vi "SLL DE Get Device Names with Catagory.vi"(8 "error in (no error)":errorcluster) -> (0 "error out":errorcluster, 2 "Devices Names":string[](array[string]), 3 "All Device Names (Chassis & Module)":cluster{"New element":tag[]}[](array[cluster]))   [LabVIEW 2009]
doc: "This VI will give all registed Device list.\nAlso this VI will giveout grouped device list for chassis and module device.\n\nCreated by Yogesh Redemptor, \nCopyright © 2008, Soliton Technologies.\nAll rights reserved."
uses:
  Program Files/National Instruments/LabVIEW 2009/resource/objmgr/daqmx.rc
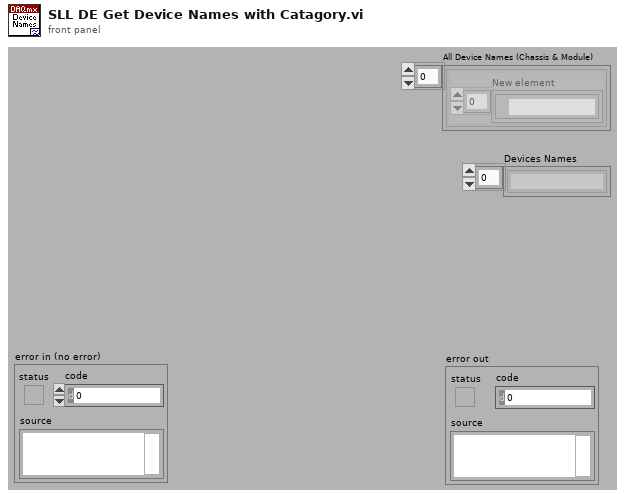
[diagram p1: front panel]
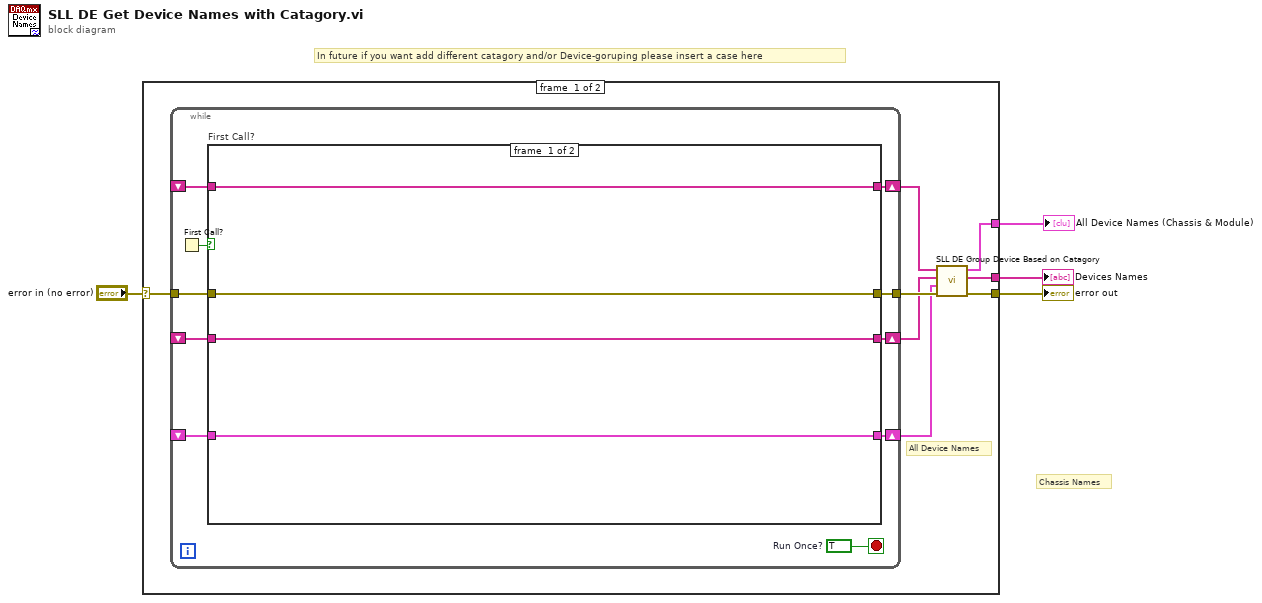
[diagram p0: block diagram]
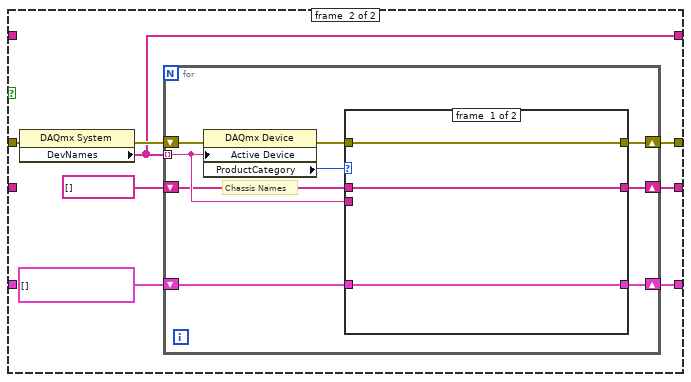
[diagram p2: hidden frame]
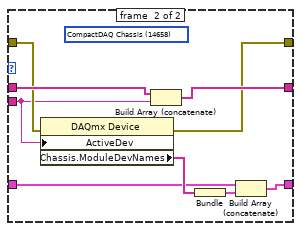
[diagram p3: hidden frame]
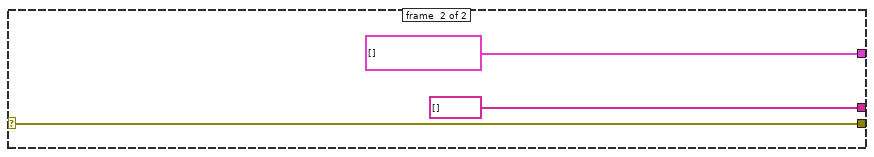
[diagram p4: hidden frame]
diagram:
  # "Chassis Names"
  # "In future if you want add different catagory and/or Device-goruping please insert a case here"
  n1 = case shown="No Error" "error in (no error)" {
    selector: "error in (no error)" -> [w12 w58]
    tunnel: [w10 w58] -> w3
    tunnel: [w6 cluster{"New element":tag[]}[] [] ("Devices after Grouping")] -> w2
    tunnel: [w5 string[] [] ("Devices Names")] -> w1
    frame #0 {
      # "All Device Names"
      n2 = while {
        tunnel: w12 -> [w22]
        tunnel: [w18] -> w11
        shift-right: [w20] -> w9
        shift-left: _ -> [w15]
        shift-right: [w19] -> w8
        shift-left: _ -> [w14]
        shift-right: [w21] -> w7
        shift-left: _ -> [w13]
        stop <- w17 stop-if-true
        w17 = TRUE  # Run Once?
        n3 = First Call?() -> (First Call?: T/F=w16:bool)
        n4 = case "First Call?" shown="True" w16 {
          tunnel: w22 -> [w25 w33]
          tunnel: [w23 w32] -> w21
          tunnel: [w26 w31] -> w20
          tunnel: [w24 w28] -> w19
          tunnel: [w25 w27] -> w18
          tunnel: w15 -> [w26 _]
          tunnel: w14 -> [w24 _]
          tunnel: w13 -> [w23 _]
          frame #0 {
          }
          frame #1 {
            n5 = property class="DAQmx System"(error in=w33) -> (error out=w34:errorcluster, "DevNames"=w31:tag[])  [unwired: 1 in, 1 out]
            n6 = for {
              tunnel: w31 -> [w41] mode=indexing
              shift-right: [w35] -> w28
              shift-left: tag[] [] -> [w40]
              shift-right: [w38] -> w27
              shift-left: w34 -> [w43]
              shift-right: [w37] -> w32
              shift-left: cluster{"Chassis.ModuleDevNames":tag[]}[] [] -> [w36]
              # "Chassis Names"
              n7 = property class="DAQmx Device"(error in=w43, "Active Device"=w41) -> (error out=w39:errorcluster, "ProductCategory"=w42:i32)  [unwired: 1 in, 1 out]
              n8 = case shown="14658" w42 {
                tunnel: w41 -> [_ w48]
                tunnel: [w45 w55] -> w35
                tunnel: w40 -> [w45 w54]
                tunnel: w39 -> [w46 w53]
                tunnel: [w46 w52] -> w38
                tunnel: [w44 w50] -> w37
                tunnel: w36 -> [w44 w49]
                frame #0 {
                }
                frame #1 {
                  (unwired) 14658 items=["M Series DAQ"=14643, "E Series DAQ"=14642, "S Series DAQ"=14644, "B Series DAQ"=14662, "SC Series DAQ"=14645, "USB DAQ"=14646, "AO Series"=14647, "Digital I/O"=14648, "TIO Series"=14661, "Dynamic Signal Acquisition"=14649, "Switches"=14650, "CompactDAQ Chassis"=14658, "C Series Module"=14659, "SCXI Module"=14660, "SCC Connector Block"=14704, "SCC Module"=14705, "NI ELVIS"=14755, "Unknown"=12588] ("ProductCategory")
                  n9 = property class="DAQmx Device"(error in=w53, "ActiveDev"=w48) -> (error out=w52:errorcluster, "Chassis.ModuleDevNames"=w51:tag[])  [unwired: 1 in, 1 out]
                  n10 = Build Array (concatenate)(w54, w48) -> (w55:tag[])
                  n11 = Bundle("Chassis.ModuleDevNames"=w51) -> (w47:cluster{"Chassis.ModuleDevNames":tag[]})  [unwired: 1 in]
                  n12 = Build Array (concatenate)(w49, w47) -> (w50:cluster{"Chassis.ModuleDevNames":tag[]}[])
                }
              }
            }
          }
        }
      }
      n13 = call "SLL DE Group Device Based on Catagory.vi"("error Input"=w11, "Module Dev Names"=w7, "Chassis Names"=w8, "Device Names"=w9) -> ("error out"=w10:errorcluster, "Devices Names"=w5:string[], "All Device Names (Chassis & Module)"=w6:cluster{"New element":tag[]}[])  [unwired: 5 in]
    }
    frame #1 {
    }
  }
  "error out" <- w3
  "All Device Names (Chassis & Module)" <- w2
  "Devices Names" <- w1
